vi "createObject.vi"(0 "HGF_Factory":refnum<class "HGF_Factory.lvclass">, 1 "objectName":string, 3 "initializationData":variant, 5 "error in (no error)":errorcluster, 6 "className":string, 7 "binaryString":string, 8 "I8 Array":i8[](array[numeric]), 9 "prependSize? (T)":bool=TRUE, 11 "byteOrder (0:big-endian, network order)":T1(ring)) -> (14 "HGF_Object":refnum<class "HGF_Factory.lvclass">, 17 "found?":bool, 19 "error out":errorcluster)   [LabVIEW 2014, in "HGF_BaseClasses.lvlib" / "HGF_Factory.lvclass"]
doc: "This VI creates initialized objects of the specified class.\n\nVariant is prefered for initialization data."
uses:
  HGF_Factory.lvclass
  HGF_Auxiliary/HGF_Auxiliary.lvlib
  HGF_Auxiliary/ErrorCode.ctl
  HGF_Auxiliary/Severity.ctl
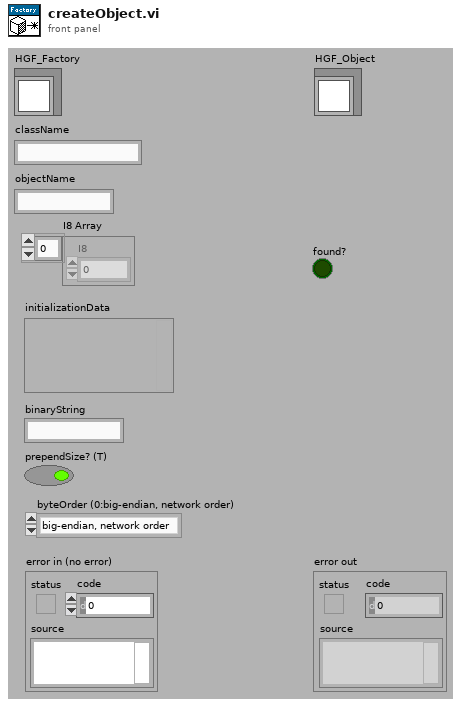
[diagram p1: front panel]
types:
  T1 = enum16{"big-endian, network order", "native, host order", "little-endian"}
  T2 = typedef "HGF_Auxiliary.lvlib/Severity.ctl" = enum16{"Info", "Warning", "Fault", "Error", "Fatal"}
  T3 = typedef "HGF_Auxiliary.lvlib/ErrorCode.ctl" = enum32{"No error", "Function not supported.", "This VI is for friends only.", "Reference object aready exisits.", "Parameter out of range.", "Not a rendezvous.", "Invalid notifier reference.", "Invalid queue reference.", "Self-Test not supported.", "Reset not supported.", "IDN query not supported.", "Error query not supported.", "Incorrect addressee.", "Object already exists.", "No class name specified", "Driver not supported", "Attribute is not writable"}
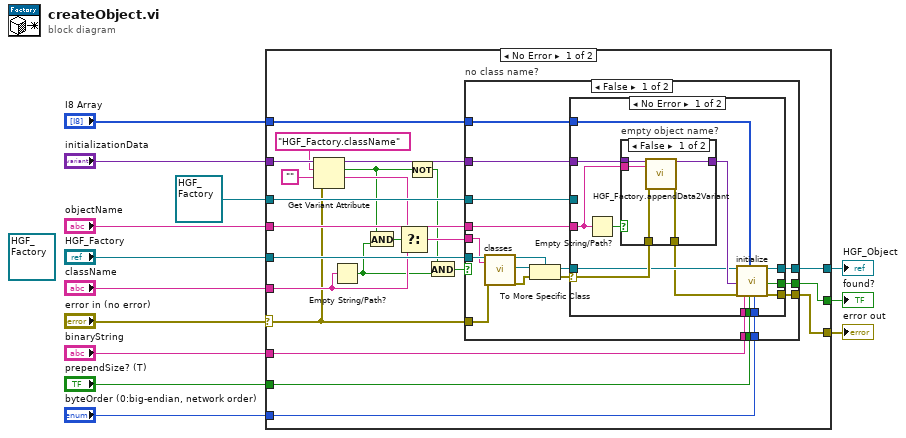
[diagram p0: block diagram]
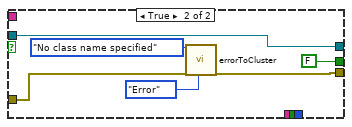
[diagram p4: hidden frame]
diagram:
  (unwired) refnum<class "HGF_Factory.lvclass"> refnum ("HGF_Factory")
  n1 = case shown="No Error" "error in (no error)" {
    selector: "error in (no error)" -> [w15 w85]
    tunnel: [w29 w85] -> w12
    tunnel: "HGF_Factory" -> [w36 _]
    tunnel: "className" -> [w21 _]
    tunnel: "I8 Array" -> [w35 _]
    tunnel: "initializationData" -> [w26 _]
    tunnel: "binaryString" -> [w34 _]
    tunnel: "prependSize? (T)" -> [w33 _]
    tunnel: "byteOrder (0:big-endian, network order)" -> [w32 _]
    tunnel: "objectName" -> [w31 _]
    tunnel: [w30 w84] -> w3
    tunnel: [w28 _] -> w2
    tunnel: refnum<class "HGF_Factory.lvclass"> refnum ("default object") -> [w27 w84]
    frame No Error {
      n2 = Get Variant Attribute(Variant=w26, name="HGF_Factory.className", default value (empty Variant)="", error in=w15) -> (duplicate Variant=w25:variant, found=w18:bool, value=w22:string)  [unwired: 1 out]
      n3 = Empty String/Path?(string/path=w21) -> (empty?=w16:bool)
      n4 = And(x=w18, y=w16) -> (x .and. y?=w19:bool)
      n5 = Select(t=w22, s=w19, f=w21) -> (s? t:f=w20:string)
      n6 = Not(x=w18) -> (.not. x?=w17:bool)
      n7 = And(x=w17, y=w16) -> (x .and. y?=w14:bool)
      n8 = case "no class name?" shown="False" w14 {
        tunnel: w36 -> [w54 w83]
        tunnel: w35 -> [w50 _]
        tunnel: w34 -> [w49 _]
        tunnel: w33 -> [w48 _]
        tunnel: w32 -> [w47 _]
        tunnel: w31 -> [w44 _]
        tunnel: [w43 w83] -> w30
        tunnel: [w42 w80] -> w29
        tunnel: [w41 FALSE ("found?")] -> w28
        tunnel: w27 -> [w40 _]
        tunnel: w25 -> [w39 _]
        tunnel: w20 -> [w38 _]
        tunnel: w15 -> [w37 w81]
        frame False {
          n9 = call-dynamic "classes.vi"("HGF_Factory"=w54, "className"=w38, "error in (no error)"=w37) -> ("HGF_Factory dup"=w51:refnum<class "HGF_Factory.lvclass">, "Object"=w53:refnum<class>, "error out"=w52:errorcluster)  [unwired: 3 in, 11 out]
          n10 = To More Specific Class(target class=w51, reference=w53, error in=w52) -> (specific class reference=w46:refnum<class "HGF_Factory.lvclass">, error out=w45:errorcluster)
          n11 = case shown="No Error" w45 {
            selector: w45 -> [w59 w77]
            tunnel: w50 -> [w66 _]
            tunnel: w39 -> [w61 _]
            tunnel: w49 -> [w62 _]
            tunnel: w48 -> [w63 _]
            tunnel: w47 -> [w64 _]
            tunnel: w46 -> [w58 _]
            tunnel: w44 -> [w56 _]
            tunnel: [w68 w76] -> w43
            tunnel: [w67 w77] -> w42
            tunnel: [w65 _] -> w41
            tunnel: w40 -> [_ w76]
            frame No Error {
              n12 = Empty String/Path?(string/path=w56) -> (empty?=w55:bool)
              n13 = case "empty object name?" shown="False" w55 {
                tunnel: w61 -> [w73 w75]
                tunnel: [w72 w75] -> w60
                tunnel: w59 -> [w71 w74]
                tunnel: [w70 w74] -> w57
                tunnel: w56 -> [w69 _]
                frame False {
                  n14 = call "HGF_Factory.appendData2Variant.vi"("initData"=w73, "objectName"=w69, "error in (no error)"=w71) -> ("dup initData"=w72:variant, "error out"=w70:errorcluster)  [unwired: 1 in, 14 out]
                }
                frame True {
                }
              }
              n15 = call-dynamic "initialize.vi"("HGF_Factory"=w58, "initializationData"=w60, "error in (no error)"=w57, "binaryString"=w62, "I8 Array"=w66, "prependSize? (T)"=w63, "byteOrder (0:big-endian, network order)"=w64) -> ("dup HGF_Factory"=w68:refnum<class "HGF_Factory.lvclass">, "found?"=w65:bool, "error out"=w67:errorcluster)  [unwired: 1 in, 9 out]
            }
            frame Error {
            }
          }
        }
        frame True {
          n16 = call "errorToCluster.vi"("error code"=ErrorCode."No class name specified", "error in (no error)"=w81, "severity (Error)"=Severity."Error") -> ("error out"=w80:errorcluster)  [unwired: 2 in, 14 out]
        }
      }
    }
    frame Error {
    }
  }
  "error out" <- w12
  "HGF_Object" <- w3
  "found?" <- w2
